vi "GVSMake DataView Idx.vi"(8 "Panel Ref Array":refnum<vi>[](array[refnum]), 9 "Spliter Ref Array":refnum<vi>[](array[refnum]), 11 "VI Ref":refnum<vi>) -> (2 "sQueueName Out":string, 3 "New DataView Idx":i32)   [LabVIEW 2013]
uses:
  Control/Graph Main Info Cluster.ctl
  GVSNew View Global.vi
  GVSView Global.vi
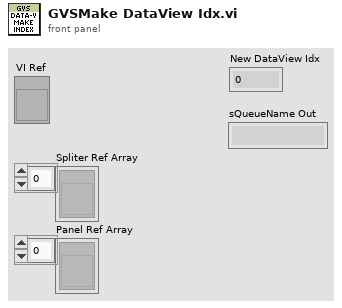
[diagram p1: front panel]
types:
  T1 = typedef "Graph Main Info Cluster.ctl" = cluster{"Selected_BarIdx":i32, "Selected_PanelIdx":i32, "Graph Main VIRef":refnum<vi>, "ToolBarClick":bool, "Spliter Ref Array":refnum<vi>[], "Panel Ref Array":refnum<vi>[], "Spliter_matrix":i32[][], "Panel_matrix":i32[][], "child_spliterIdx_matrix":i32[][], "split_pos_matrix":i32[][], "Title State":bool, "sQueueName":string, "Frame nID":i32, "Graph VIRef Array":cluster{"Graph VIRef":refnum<vi>, "Panel Idx":i32, "Frame VIRef":refnum<vi>, "Icon Ring":i32, "Graph Type":string}[], "View Type":string}
  T2 = cluster{"sAction":string, "sType":string, "sQueueName":string, "sGraphName":string, "sData":string, "nData":i32, "pVIRef":refnum<vi>, "pSPRef":refnum<vi>}
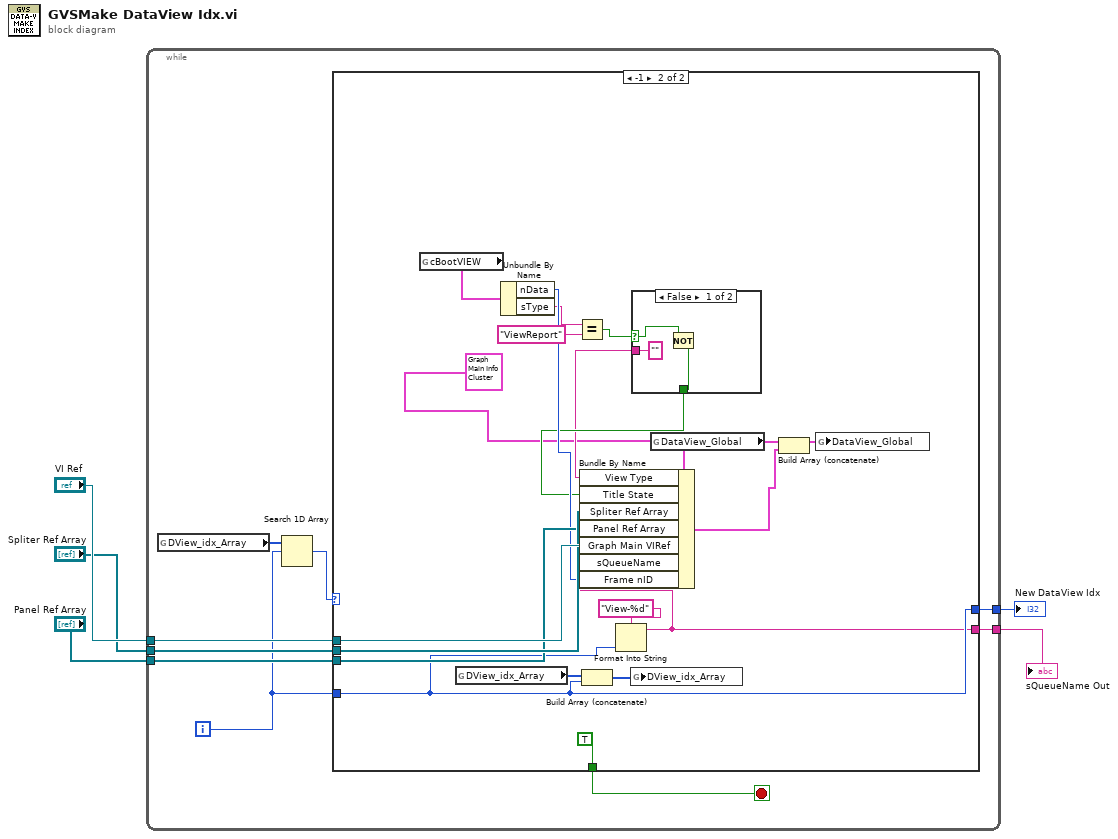
[diagram p0: block diagram]
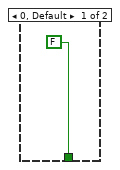
[diagram p2: hidden frame]
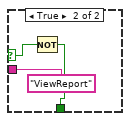
[diagram p3: hidden frame]
diagram:
  n1 = while {
    tunnel: [w11] -> w5
    tunnel: "VI Ref" -> [w10]
    tunnel: "Spliter Ref Array" -> [w9]
    tunnel: "Panel Ref Array" -> [w8]
    tunnel: [w7] -> w1
    i -> [w6]
    stop <- w12 stop-if-true
    n2 = global read "GVSNew View Global.vi" "DView_idx_Array"() -> (w14:i32[])
    n3 = Search 1D Array(1D array=w14, element=w6) -> (index of element=w13:i32)  [unwired: 1 in]
    n4 = case shown="-1" w13 {
      tunnel: w6 -> [_ w28]
      tunnel: [FALSE TRUE] -> w12
      tunnel: [_ w28] -> w11
      tunnel: w10 -> [_ w32]
      tunnel: w9 -> [_ w31]
      tunnel: w8 -> [_ w30]
      tunnel: [_ w27] -> w7
      frame 0, Default {
      }
      frame -1 {
        n5 = global read "GVSView Global.vi" "cBootVIEW"() -> (w23:T2)
        n6 = global read "GVSNew View Global.vi" "DView_idx_Array"() -> (w35:i32[])
        n7 = Unbundle By Name(w23) -> ("nData"=w22:i32, "sType"=w21:string)
        n8 = Equal?(x=w21, y="ViewReport") -> (x = y?=w17:bool)
        n9 = Build Array (concatenate)(w35, w28) -> (w34:i32[])
        n10 = Format Into String(format string="View-%d", w28) -> (resulting string=w27:string)  [unwired: 2 in, 1 out]
        n11 = global write "GVSNew View Global.vi" "DView_idx_Array"(w34) -> ()
        n12 = case shown="False" w17 {
          selector: w17 -> [w37 w39]
          tunnel: [w36 w41] -> w19
          tunnel: ["" ("View Type") "ViewReport" ("View Type")] -> w18
          frame False {
            n13 = Not(x=w37) -> (.not. x?=w36:bool)
          }
          frame True {
            n14 = Not(x=w39) -> (.not. x?=w41:bool)
          }
        }
        n15 = Bundle By Name(cluster=T1 {"Selected_BarIdx"=0, "Selected_PanelIdx"=0, "Graph Main VIRef"=refnum, "ToolBarClick"=FALSE, "Spliter Ref Array"=[], "Panel Ref Array"=[], "Spliter_matrix"=[], "Panel_matrix"=[[-1], [0], [-1]], "child_spliterIdx_matrix"=[[0, 0, 0, 0, 0, 0, 0, 0, 0, 0, 0, 0, 0, 0, 0, 0, 0, 0, 0, 0, 0, 0, 0, 0, 0, 0, 0, 0, 0, 0, 0], [0, 0, 0, 0, 0, 0, 0, 0, 0, 0, 0, 0, 0, 0, 0, 0, 0, 0, 0, 0, 0, 0, 0, 0, 0, 0, 0, 0, 0, 0, 0], [0, 0, 0, 0, 0, 0, 0, 0, 0, 0, 0, 0, 0, 0, 0, 0, 0, 0, 0, 0, 0, 0, 0, 0, 0, 0, 0, 0, 0, 0, 0], [0, 0, 0, 0, 0, 0, 0, 0, 0, 0, 0, 0, 0, 0, 0, 0, 0, 0, 0, 0, 0, 0, 0, 0, 0, 0, 0, 0, 0, 0, 0], [0, 0, 0, 0, 0, 0, 0, 0, 0, 0, 0, 0, 0, 0, 0, 0, 0, 0, 0, 0, 0, 0, 0, 0, 0, 0, 0, 0, 0, 0, 0], [0, 0, 0, 0, 0, 0, 0, 0, 0, 0, 0, 0, 0, 0, 0, 0, 0, 0, 0, 0, 0, 0, 0, 0, 0, 0, 0, 0, 0, 0, 0], [0, 0, 0, 0, 0, 0, 0, 0, 0, 0, 0, 0, 0, 0, 0, 0, 0, 0, 0, 0, 0, 0, 0, 0, 0, 0, 0, 0, 0, 0, 0], [0, 0, 0, 0, 0, 0, 0, 0, 0, 0, 0, 0, 0, 0, 0, 0, 0, 0, 0, 0, 0, 0, 0, 0, 0, 0, 0, 0, 0, 0, 0], [0, 0, 0, 0, 0, 0, 0, 0, 0, 0, 0, 0, 0, 0, 0, 0, 0, 0, 0, 0, 0, 0, 0, 0, 0, 0, 0, 0, 0, 0, 0], [0, 0, 0, 0, 0, 0, 0, 0, 0, 0, 0, 0, 0, 0, 0, 0, 0, 0, 0, 0, 0, 0, 0, 0, 0, 0, 0, 0, 0, 0, 0], [0, 0, 0, 0, 0, 0, 0, 0, 0, 0, 0, 0, 0, 0, 0, 0, 0, 0, 0, 0, 0, 0, 0, 0, 0, 0, 0, 0, 0, 0, 0], [0, 0, 0, 0, 0, 0, 0, 0, 0, 0, 0, 0, 0, 0, 0, 0, 0, 0, 0, 0, 0, 0, 0, 0, 0, 0, 0, 0, 0, 0, 0], [0, 0, 0, 0, 0, 0, 0, 0, 0, 0, 0, 0, 0, 0, 0, 0, 0, 0, 0, 0, 0, 0, 0, 0, 0, 0, 0, 0, 0, 0, 0], [0, 0, 0, 0, 0, 0, 0, 0, 0, 0, 0, 0, 0, 0, 0, 0, 0, 0, 0, 0, 0, 0, 0, 0, 0, 0, 0, 0, 0, 0, 0], [0, 0, 0, 0, 0, 0, 0, 0, 0, 0, 0, 0, 0, 0, 0, 0, 0, 0, 0, 0, 0, 0, 0, 0, 0, 0, 0, 0, 0, 0, 0], [0, 0, 0, 0, 0, 0, 0, 0, 0, 0, 0, 0, 0, 0, 0, 0, 0, 0, 0, 0, 0, 0, 0, 0, 0, 0, 0, 0, 0, 0, 0], [0, 0, 0, 0, 0, 0, 0, 0, 0, 0, 0, 0, 0, 0, 0, 0, 0, 0, 0, 0, 0, 0, 0, 0, 0, 0, 0, 0, 0, 0, 0], [0, 0, 0, 0, 0, 0, 0, 0, 0, 0, 0, 0, 0, 0, 0, 0, 0, 0, 0, 0, 0, 0, 0, 0, 0, 0, 0, 0, 0, 0, 0], [0, 0, 0, 0, 0, 0, 0, 0, 0, 0, 0, 0, 0, 0, 0, 0, 0, 0, 0, 0, 0, 0, 0, 0, 0, 0, 0, 0, 0, 0, 0], [0, 0, 0, 0, 0, 0, 0, 0, 0, 0, 0, 0, 0, 0, 0, 0, 0, 0, 0, 0, 0, 0, 0, 0, 0, 0, 0, 0, 0, 0, 0], [0, 0, 0, 0, 0, 0, 0, 0, 0, 0, 0, 0, 0, 0, 0, 0, 0, 0, 0, 0, 0, 0, 0, 0, 0, 0, 0, 0, 0, 0, 0], [0, 0, 0, 0, 0, 0, 0, 0, 0, 0, 0, 0, 0, 0, 0, 0, 0, 0, 0, 0, 0, 0, 0, 0, 0, 0, 0, 0, 0, 0, 0], [0, 0, 0, 0, 0, 0, 0, 0, 0, 0, 0, 0, 0, 0, 0, 0, 0, 0, 0, 0, 0, 0, 0, 0, 0, 0, 0, 0, 0, 0, 0], [0, 0, 0, 0, 0, 0, 0, 0, 0, 0, 0, 0, 0, 0, 0, 0, 0, 0, 0, 0, 0, 0, 0, 0, 0, 0, 0, 0, 0, 0, 0], [0, 0, 0, 0, 0, 0, 0, 0, 0, 0, 0, 0, 0, 0, 0, 0, 0, 0, 0, 0, 0, 0, 0, 0, 0, 0, 0, 0, 0, 0, 0], [0, 0, 0, 0, 0, 0, 0, 0, 0, 0, 0, 0, 0, 0, 0, 0, 0, 0, 0, 0, 0, 0, 0, 0, 0, 0, 0, 0, 0, 0, 0], [0, 0, 0, 0, 0, 0, 0, 0, 0, 0, 0, 0, 0, 0, 0, 0, 0, 0, 0, 0, 0, 0, 0, 0, 0, 0, 0, 0, 0, 0, 0], [0, 0, 0, 0, 0, 0, 0, 0, 0, 0, 0, 0, 0, 0, 0, 0, 0, 0, 0, 0, 0, 0, 0, 0, 0, 0, 0, 0, 0, 0, 0], [0, 0, 0, 0, 0, 0, 0, 0, 0, 0, 0, 0, 0, 0, 0, 0, 0, 0, 0, 0, 0, 0, 0, 0, 0, 0, 0, 0, 0, 0, 0], [0, 0, 0, 0, 0, 0, 0, 0, 0, 0, 0, 0, 0, 0, 0, 0, 0, 0, 0, 0, 0, 0, 0, 0, 0, 0, 0, 0, 0, 0, 0], [0, 0, 0, 0, 0, 0, 0, 0, 0, 0, 0, 0, 0, 0, 0, 0, 0, 0, 0, 0, 0, 0, 0, 0, 0, 0, 0, 0, 0, 0, 0]], "split_pos_matrix"=[], "Title State"=FALSE, "sQueueName"="", "Frame nID"=0, "Graph VIRef Array"=[], "View Type"=""} ("Cluster"), "View Type"=w18, "Title State"=w19, "Spliter Ref Array"=w31, "Panel Ref Array"=w30, "Graph Main VIRef"=w32, "sQueueName"=w27, "Frame nID"=w22) -> (w24:T1)
        n16 = global read "GVSNew View Global.vi" "DataView_Global"() -> (w26:T1[])
        n17 = Build Array (concatenate)(w26, w24) -> (w25:T1[])
        n18 = global write "GVSNew View Global.vi" "DataView_Global"(w25) -> ()
      }
    }
  }
  "New DataView Idx" <- w5
  "sQueueName Out" <- w1
